vi "FTW-Message-Multipart-Interpret.vi"(0 "FTW Message":refnum<class "FTW-Message.lvclass">, 11 "error in":errorcluster) -> (4 "FTW Message out":refnum<class "FTW-Message.lvclass">, 6 "Message":T1, 15 "error out":errorcluster)   [LabVIEW 2013, in "FTW-Message.lvclass"]
uses:
  FTW-Message.lvclass
  Payload/FTW-MessagePayload.ctl
  FTW-Message.lvclass/FTW-Message.ctl
panel:
  # "Inputs"
  # "Outputs"
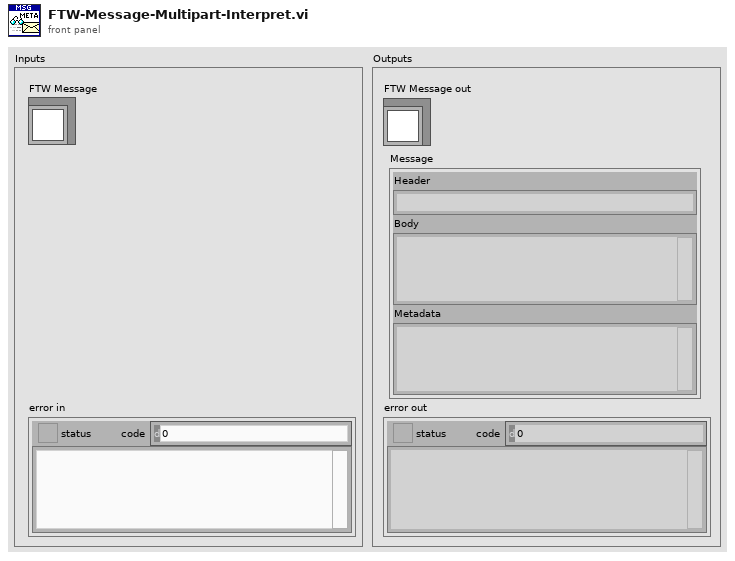
[diagram p1: front panel]
types:
  T1 = typedef "FTW-MessagePayload.ctl" = cluster{"Header":string, "Body":string, "Metadata":string}
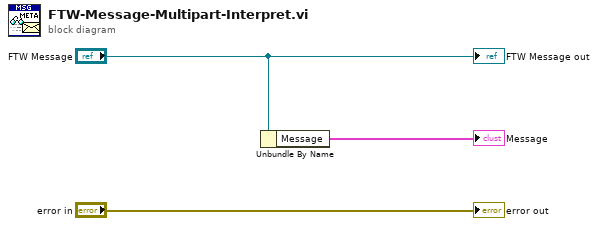
[diagram p0: block diagram]
diagram:
  n1 = Unbundle By Name("FTW Message") -> ("Message"=→"Message":T1)
  "error out" <- "error in"
  "FTW Message out" <- "FTW Message"
